vi "Complex LU Factorization.vi"(0 "A":T1) -> (1 "L":T1, 2 "U":T1, 3 "P":i32[][](array[numeric]), 4 "error":i32)   [LabVIEW 2020, in "NI_AALPro.lvlib"]
doc: "Performs the LU factorization of <B>A</B> so that <B>PA</B> = <B>LU</B>. Wire data to the <B>A</B> input to determine the polymorphic instance to use or manually select the instance."
uses:
  <vilib>/Analysis/NI_AALPro.lvlib
  <vilib>/Analysis/Matrix/Datatypes/ComplexMatrix.ctl
  <vilib>/Analysis/NI_AALBase.lvlib
  <vilib>/Analysis/Matrix/NI_Matrix.lvlib
panel:
  # "Complex LU Factorization"
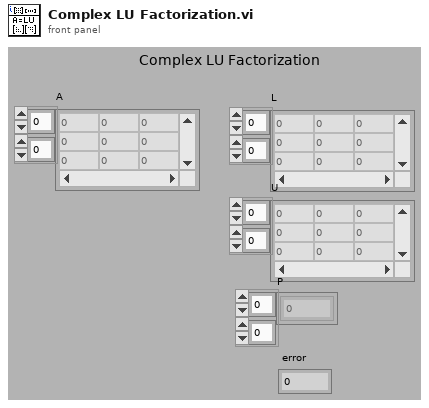
[diagram p1: front panel]
types:
  T1 = typedef "NI_Matrix.lvlib/ComplexMatrix.ctl" = cdb[][]
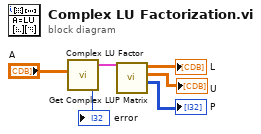
[diagram p0: block diagram]
diagram:
  n1 = call <vilib>:"Complex LU Factor.vi"("A"="A") -> ("LU Info"=w1:cluster{"LU":cdb[][], "Pivot":i32[]}, "error"=→"error":i32)  [unwired: 1 out]
  n2 = call <vilib>:"Get Complex LUP Matrix.vi"("LU Info"=w1) -> ("L"=→"L":T1, "U"=→"U":T1, "P"=→"P":i32[][])  [unwired: 1 in]
